vi "mechanical_mode.vi"(6 "C4":fxp<+/-,32,1>=0.999985234811902, 7 "reset":bool=TRUE, 8 "input valid":bool=TRUE, 9 "C5":fxp<+/-,48,-16>=-5.4794710435679406e-14, 10 "C3":fxp<+/-,48,18>=-2.180195599794388, 11 "sqV":fxp<+/-,64,32>) -> (0 "output valid":bool, 3 "W1(n)*dt":fxp<+/-,64,0>)   [LabVIEW 2018]
uses:
  <vilib>/rvi/FXPMathLib/FxpMul/XNode/nifxpmath_Multiplier.xnode
  <vilib>/rvi/FXPMathLib/FxpAdd/XNode/nifxpmath_Add.xnode
  <vilib>/rvi/FXPMathLib/sim/FxpSim.dll
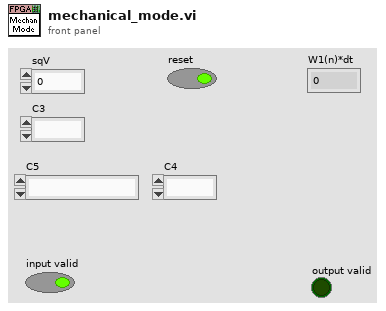
[diagram p1: front panel]
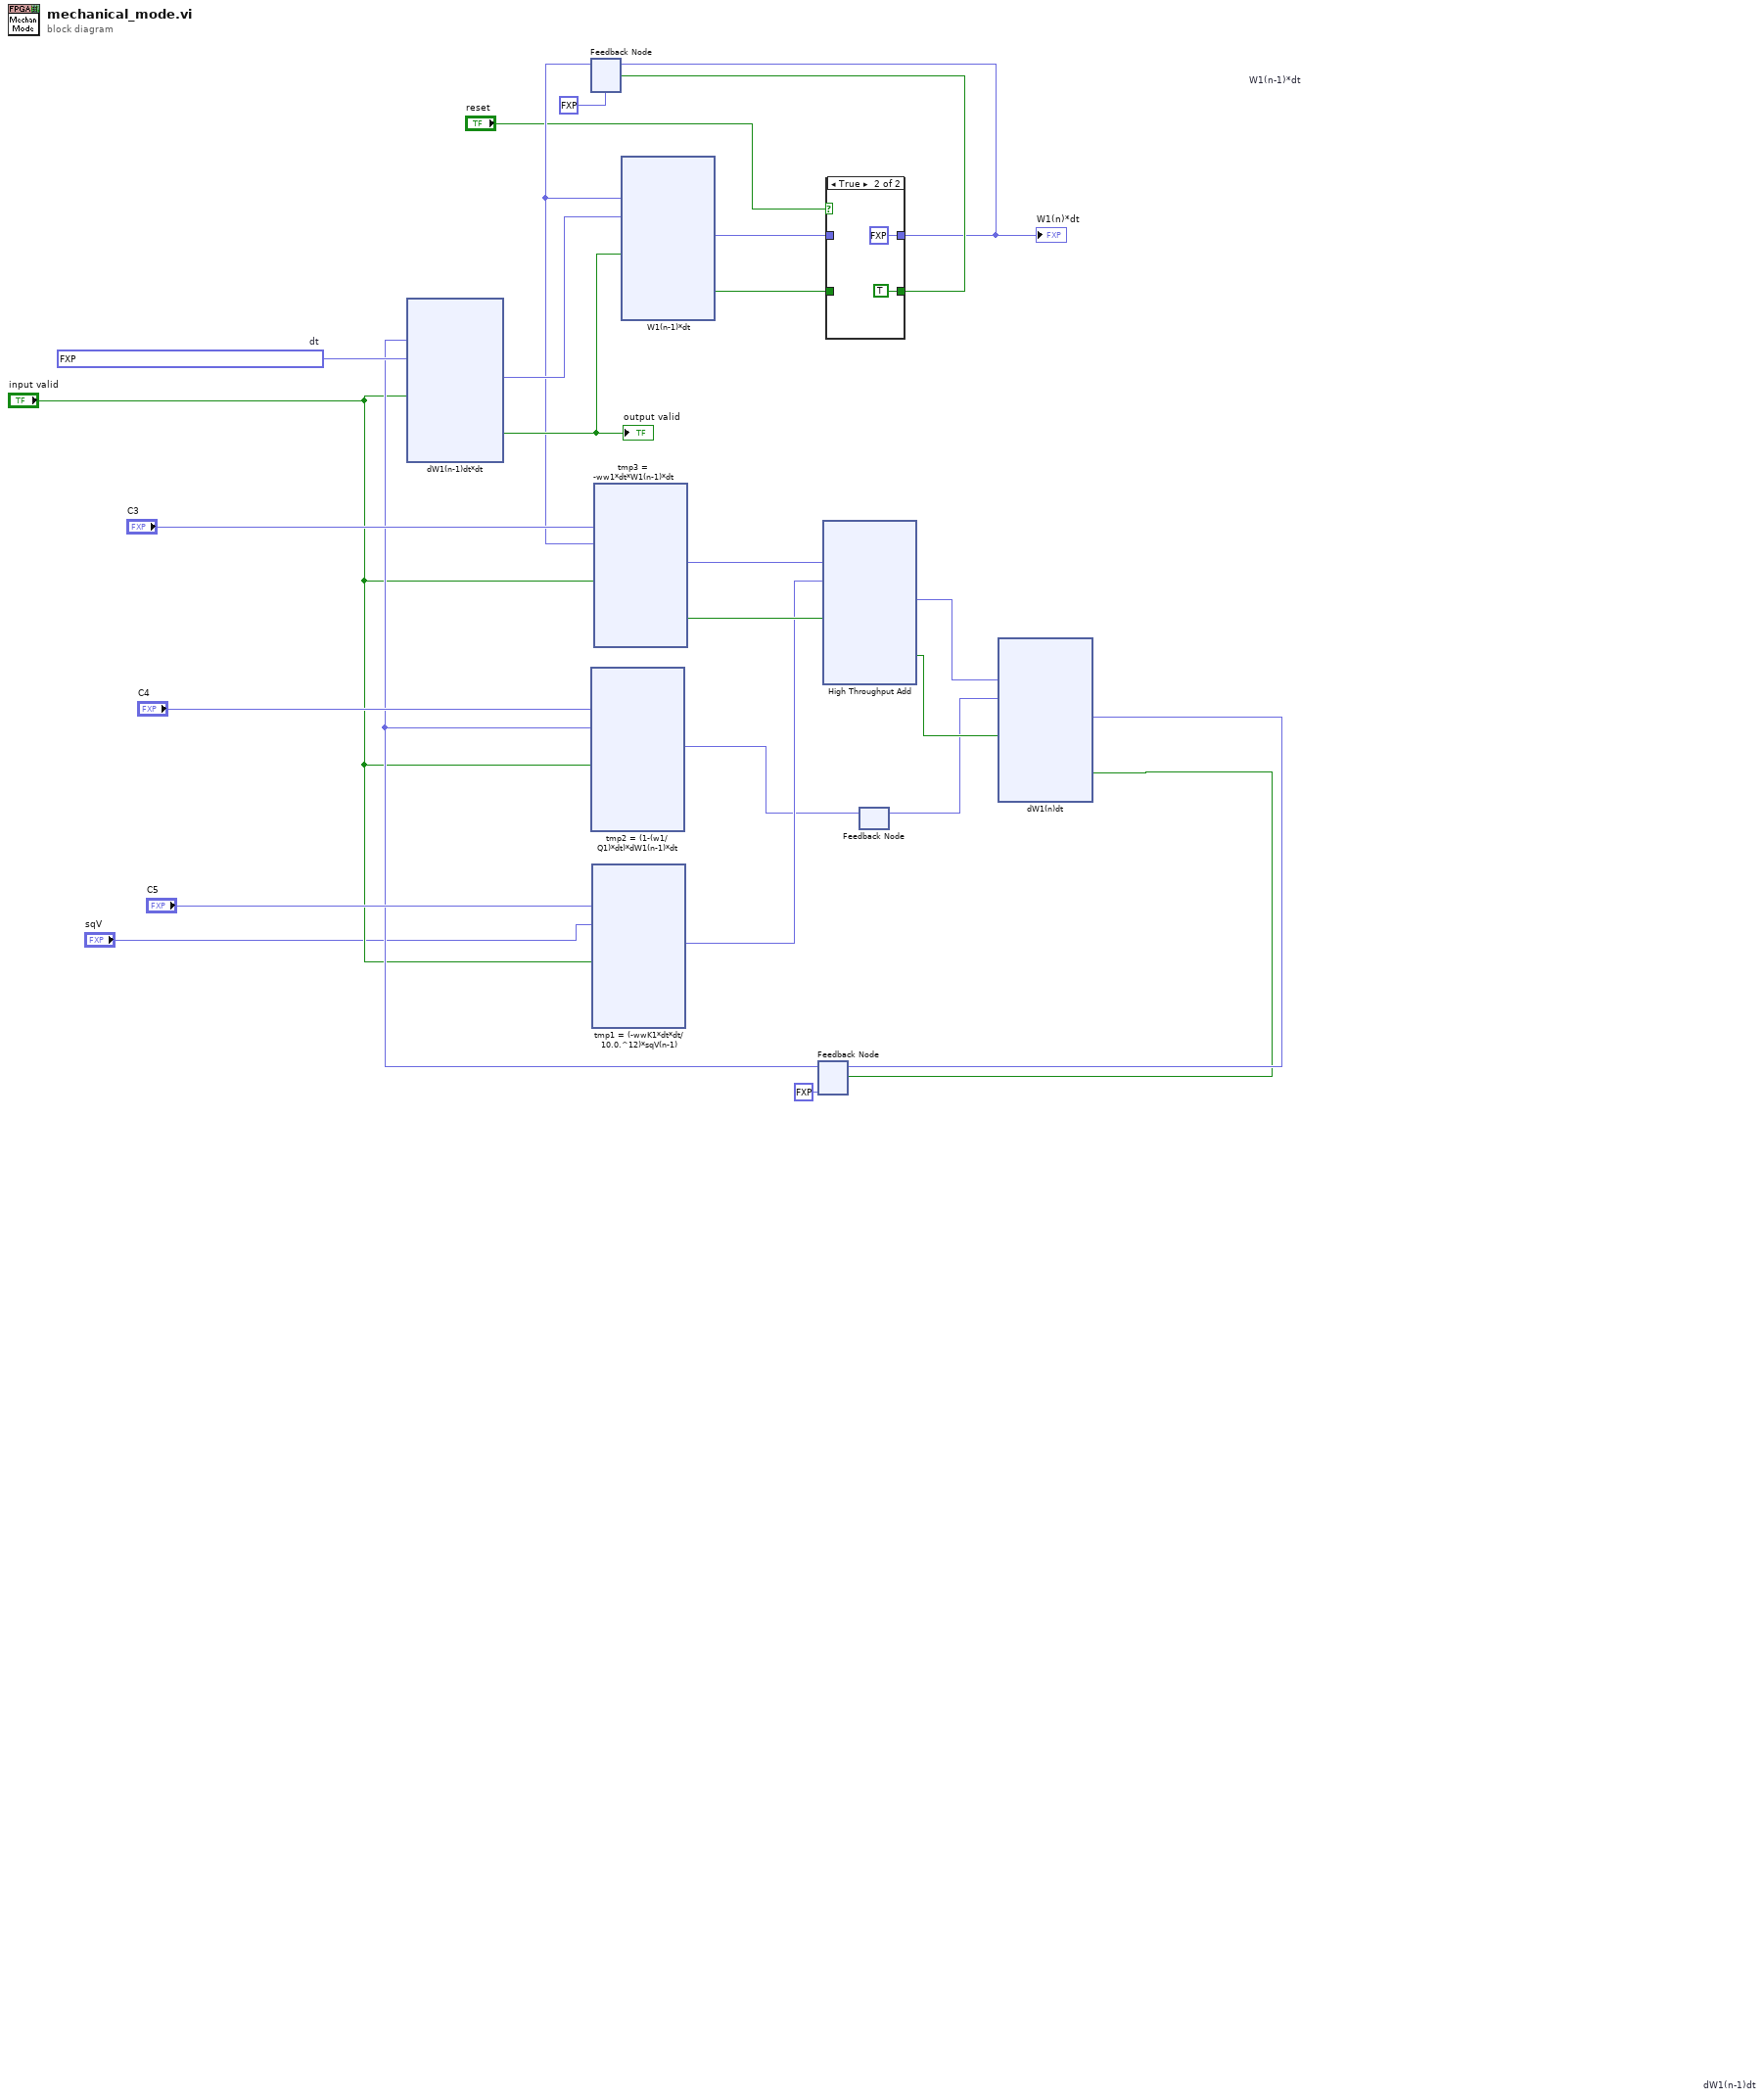
[diagram p0: block diagram]
diagram:
  w25 = fxp<+/-,32,-16> 1.0000000116860974e-07  # dt
  n1 = feedback #1 "W1(n-1)*dt"(fxp<+/-,64,0> 0.0 ("dt")) -> (w6:fxp<+/-,64,0>)
  n2 = xnode "tmp1 = (-wwK1*dt*dt/10.0.^12)*sqV(n-1)"("x"="C5", "y"="sqV", "input valid"="input valid") -> ("x*y"=w14:fxp<+/-,64,-4>)  [unwired: 1 in, 2 out]
  n3 = xnode "tmp3 = -ww1*dt*W1(n-1)*dt"("x"="C3", "y"=w6, "input valid"="input valid") -> ("x*y"=w15:fxp<+/-,64,-4>, "output valid"=w21:bool)  [unwired: 1 in, 1 out]
  n4 = feedback #2 "dW1(n-1)dt"(fxp<+/-,64,10> 0.0 ("x")) -> (w18:fxp<+/-,64,10>)
  n5 = xnode "dW1(n-1)dt*dt"("x"=w18, "y"=w25, "input valid"="input valid") -> ("x*y"=w7:fxp<+/-,64,-16>, "output valid"=w8:bool)  [unwired: 1 in, 1 out]
  "output valid" <- w8
  n6 = xnode "tmp2 = (1-(w1/Q1)*dt)*dW1(n-1)*dt"("x"="C4", "y"=w18, "input valid"="input valid") -> ("x*y"=w13:fxp<+/-,64,10>)  [unwired: 1 in, 2 out]
  n7 = xnode "W1(n-1)*dt"("x"=w6, "y"=w7, "input valid"=w8) -> ("x+y"=w5:fxp<+/-,64,0>, "output valid"=w3:bool)  [unwired: 1 in, 1 out]
  n8 = xnode ("High Throughput Add")("x"=w15, "y"=w14, "input valid"=w21) -> ("x+y"=w19:fxp<+/-,64,-2>, "output valid"=w20:bool)  [unwired: 1 in, 1 out]
  n9 = case shown="True" "reset" {
    tunnel: w5 -> [w28 _]
    tunnel: w3 -> [w27 _]
    tunnel: [w28 fxp<+/-,64,0> 0.0 ("x+y")] -> w1
    tunnel: [w27 TRUE ("output valid")] -> w2
    frame False {
    }
    frame True {
    }
  }
  "W1(n)*dt" <- w1
  n10 = feedback-in #1(w1, w2) -> ()
  n11 = feedback #3() -> (w16:fxp<+/-,64,10>)  [unwired: 1 in]
  n12 = feedback-in #3(w13) -> ()
  n13 = xnode "dW1(n)dt"("x"=w19, "y"=w16, "input valid"=w20) -> ("x+y"=w12:fxp<+/-,64,10>, "output valid"=w11:bool)  [unwired: 1 in, 1 out]
  n14 = feedback-in #2(w12, w11) -> ()
